vi "Configure AC Filter.vi"(8 "error in (no error)":errorcluster, 9 "Maximum Frequency(2000 Hz)":dbl=2000.0, 10 "Minimum Frequency(20 Hz)":dbl=20.0, 11 "VISA resource name":refnum<visa-resource-name>) -> (0 "error out":errorcluster, 3 "VISA resource name out":refnum<visa-resource-name>)   [LabVIEW 2020, in "Agilent 3458.lvlib"]
doc: "Configures the lowest frequency and highest frequency bandwidths for AC measurements."
uses:
  Agilent 3458.lvlib
panel:
  # "AC Filter Bandwidth"
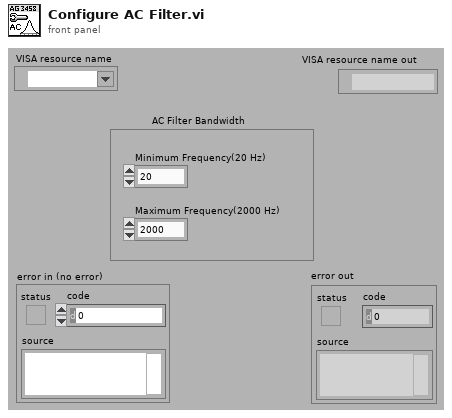
[diagram p1: front panel]
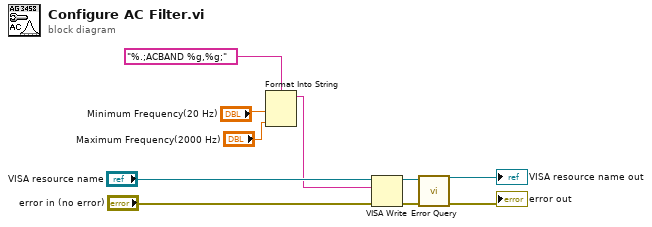
[diagram p0: block diagram]
diagram:
  n1 = Format Into String(format string="%.;ACBAND %g,%g;", "Minimum Frequency(20 Hz)", "Maximum Frequency(2000 Hz)") -> (resulting string=w2:string)  [unwired: 2 in, 1 out]
  n2 = VISA Write(VISA resource name="VISA resource name", write buffer=w2, error in (no error)="error in (no error)") -> (VISA resource name out=w8:refnum<visa-resource-name>, error out=w9:errorcluster)  [unwired: 1 out]
  n3 = call "Error Query.vi"("error in (no error)"=w9, "VISA resource name"=w8) -> ("error out"=→"error out":errorcluster, "VISA resource name out"=→"VISA resource name out":refnum<visa-resource-name>)  [unwired: 6 in, 2 out]
